vi "Corr Digitizer to Meas Header.vi"(8 "error in":errorcluster, 11 "digitizer in":T1) -> (0 "error out":errorcluster, 2 "info data out":string, 3 "digitizer out":T1)   [LabVIEW 2013]
doc: "This VI will copy digitizer corrections to the measurement INFO header."
uses:
  Corr Digitizers.ctl
  octave/infolib.lvlibp/Private/Add key polymorph parts/String.vi
  octave/infolib.lvlibp
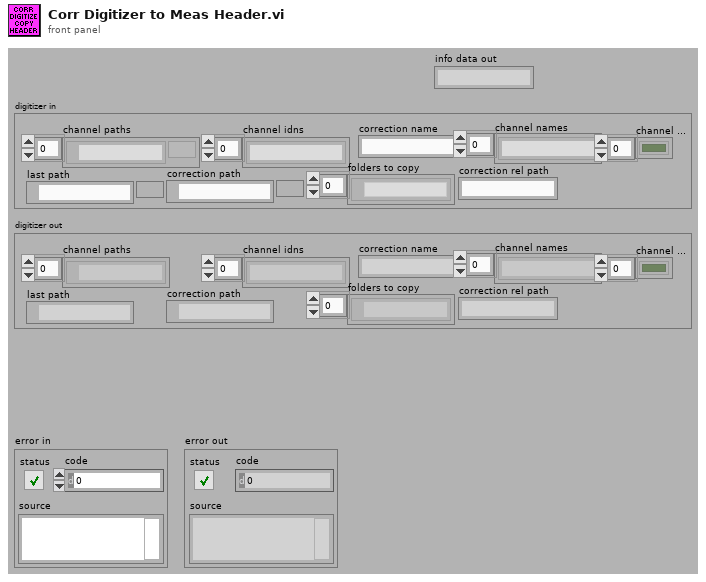
[diagram p1: front panel]
types:
  T1 = typedef "Corr Digitizers.ctl" = cluster{"last path":path, "channel paths":path[], "channel idns":string[], "correction name":string, "channel names":string[], "folders to copy":path[], "channel valid":bool[], "correction path":path, "correction rel path":string}
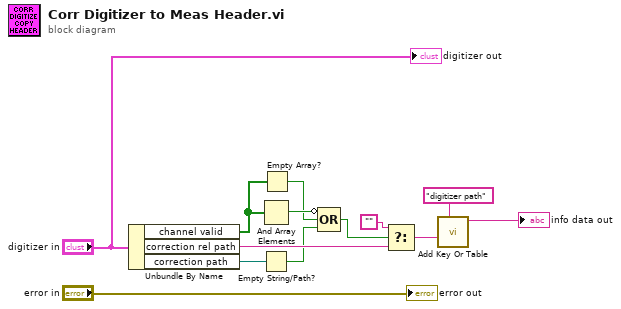
[diagram p0: block diagram]
diagram:
  n1 = Unbundle By Name("digitizer in") -> ("channel valid"=w2:bool[], "correction rel path"=w8:string, "correction path"=w9:path)
  n2 = And Array Elements(Boolean array=w2) -> (logical AND=w4:bool)
  n3 = Empty String/Path?(string/path=w9) -> (empty?=w3:bool)
  n4 = Empty Array?(array=w2) -> (empty?=w1:bool)
  n5 = Compound Arithmetic op=OR(invert w4, w1, w3) -> (w5:bool)
  n6 = Select(t="", s=w5, f=w8) -> (s? t:f=w6:string)
  n7 = call-poly "Add Key Or Table.vi"("key description"="digitizer path", "string"=w6) -> ("info data out"=→"info data out":string)  [unwired: 8 in, 1 out]
  "error out" <- "error in"
  "digitizer out" <- "digitizer in"
